vi "CurrentShiftCalc.vi"(8 "Date/Time":string, 9 "3rdShiftConfig":T1={"StartHour"=[{"Hour"=5, "Minute"=0}, {"Hour"=6, "Minute"=0}, {"Hour"=7, "Minute"=0}, {"Hour"=7, "Minute"=30}, {"Hour"=0, "Minute"=0}, {"Hour"=0, "Minute"=0}, {"Hour"=0, "Minute"=0}, {"Hour"=0, "Minute"=0}, {"Hour"=0, "Minute"=0}], "Goal"=[], "EndHour"=[{"Hour"=5, "Minute"=59}, {"Hour"=6, "Minute"=59}, {"Hour"=7, "Minute"=10}, {"Hour"=7, "Minute"=59}, {"Hour"=0, "Minute"=0}, {"Hour"=0, "Minute"=0}, {"Hour"=0, "Minute"=0}, {"Hour"=0, "Minute"=0}, {"Hour"=0, "Minute"=0}], "AM/PM"=[]} caption="3rdShift" {"AM/PM"."AM/PM" items=["AM", "PM"]; "EndHour"."Minute" items=["00", "1", "2", "3", "4", "5", "6", "7", "8", "9", "10", "11", "12", "13", "14", "15", "16", "17", "18", "19", "20", "21", "22", "23", "24", "25", "26", "27", "28", "29", "30", "31", "32", "33", "34", "35", "36", "37", "38", "39", "40", "41", "42", "43", "44", "45", "46", "47", "48", "49", "50", "51", "52", "53", "54", "55", "56", "57", "58", "59"]; "EndHour"."Hour" items=["0", "1", "2", "3", "4", "5", "6", "7", "8", "9", "10", "11", "12", "13", "14", "15", "16", "17", "18", "19", "20", "21", "22", "23"]; "StartHour"."Minute" items=["00", "1", "2", "3", "4", "5", "6", "7", "8", "9", "10", "11", "12", "13", "14", "15", "16", "17", "18", "19", "20", "21", "22", "23", "24", "25", "26", "27", "28", "29", "30", "31", "32", "33", "34", "35", "36", "37", "38", "39", "40", "41", "42", "43", "44", "45", "46", "47", "48", "49", "50", "51", "52", "53", "54", "55", "56", "57", "58", "59"]; "StartHour"."Hour" items=["0", "1", "2", "3", "4", "5", "6", "7", "8", "9", "10", "11", "12", "13", "14", "15", "16", "17", "18", "19", "20", "21", "22", "23"]}, 10 "2ndShiftConfig":T1={"StartHour"=[{"Hour"=5, "Minute"=0}, {"Hour"=6, "Minute"=0}, {"Hour"=7, "Minute"=0}, {"Hour"=7, "Minute"=30}, {"Hour"=0, "Minute"=0}, {"Hour"=0, "Minute"=0}, {"Hour"=0, "Minute"=0}, {"Hour"=0, "Minute"=0}, {"Hour"=0, "Minute"=0}], "Goal"=[], "EndHour"=[{"Hour"=5, "Minute"=59}, {"Hour"=6, "Minute"=59}, {"Hour"=7, "Minute"=10}, {"Hour"=7, "Minute"=59}, {"Hour"=0, "Minute"=0}, {"Hour"=0, "Minute"=0}, {"Hour"=0, "Minute"=0}, {"Hour"=0, "Minute"=0}, {"Hour"=0, "Minute"=0}], "AM/PM"=[{"AM/PM"=1}, {"AM/PM"=1}, {"AM/PM"=1}, {"AM/PM"=1}, {"AM/PM"=1}, {"AM/PM"=1}, {"AM/PM"=1}, {"AM/PM"=1}, {"AM/PM"=1}]} caption="2ndShift" {"AM/PM"."AM/PM" items=["AM", "PM"]; "EndHour"."Minute" items=["00", "1", "2", "3", "4", "5", "6", "7", "8", "9", "10", "11", "12", "13", "14", "15", "16", "17", "18", "19", "20", "21", "22", "23", "24", "25", "26", "27", "28", "29", "30", "31", "32", "33", "34", "35", "36", "37", "38", "39", "40", "41", "42", "43", "44", "45", "46", "47", "48", "49", "50", "51", "52", "53", "54", "55", "56", "57", "58", "59"]; "EndHour"."Hour" items=["00", "1", "2", "3", "4", "5", "6", "7", "8", "9", "10", "11", "12", "13", "14", "15", "16", "17", "18", "19", "20", "21", "22", "23"]; "StartHour"."Minute" items=["00", "1", "2", "3", "4", "5", "6", "7", "8", "9", "10", "11", "12", "13", "14", "15", "16", "17", "18", "19", "20", "21", "22", "23", "24", "25", "26", "27", "28", "29", "30", "31", "32", "33", "34", "35", "36", "37", "38", "39", "40", "41", "42", "43", "44", "45", "46", "47", "48", "49", "50", "51", "52", "53", "54", "55", "56", "57", "58", "59"]; "StartHour"."Hour" items=["0", "1", "2", "3", "4", "5", "6", "7", "8", "9", "10", "11", "12", "13", "14", "15", "16", "17", "18", "19", "20", "21", "22", "23"]}, 11 "1stShiftConfig":T1={"StartHour"=[{"Hour"=5, "Minute"=0}, {"Hour"=6, "Minute"=0}, {"Hour"=7, "Minute"=0}, {"Hour"=7, "Minute"=30}, {"Hour"=0, "Minute"=0}, {"Hour"=0, "Minute"=0}, {"Hour"=0, "Minute"=0}, {"Hour"=0, "Minute"=0}, {"Hour"=0, "Minute"=0}], "Goal"=[], "EndHour"=[{"Hour"=5, "Minute"=59}, {"Hour"=6, "Minute"=59}, {"Hour"=7, "Minute"=10}, {"Hour"=7, "Minute"=59}, {"Hour"=0, "Minute"=0}, {"Hour"=0, "Minute"=0}, {"Hour"=0, "Minute"=0}, {"Hour"=0, "Minute"=0}, {"Hour"=0, "Minute"=0}], "AM/PM"=[{"AM/PM"=0}, {"AM/PM"=0}, {"AM/PM"=0}, {"AM/PM"=0}, {"AM/PM"=0}, {"AM/PM"=0}, {"AM/PM"=0}, {"AM/PM"=0}, {"AM/PM"=0}]} caption="1stShift" {"AM/PM"."AM/PM" items=["AM", "PM"]; "EndHour"."Minute" items=["00", "1", "2", "3", "4", "5", "6", "7", "8", "9", "10", "11", "12", "13", "14", "15", "16", "17", "18", "19", "20", "21", "22", "23", "24", "25", "26", "27", "28", "29", "30", "31", "32", "33", "34", "35", "36", "37", "38", "39", "40", "41", "42", "43", "44", "45", "46", "47", "48", "49", "50", "51", "52", "53", "54", "55", "56", "57", "58", "59"]; "EndHour"."Hour" items=["0", "1", "2", "3", "4", "5", "6", "7", "8", "9", "10", "11", "12", "13", "14", "15", "16", "17", "18", "19", "20", "21", "22", "23"]; "StartHour"."Minute" items=["00", "1", "2", "3", "4", "5", "6", "7", "8", "9", "10", "11", "12", "13", "14", "15", "16", "17", "18", "19", "20", "21", "22", "23", "24", "25", "26", "27", "28", "29", "30", "31", "32", "33", "34", "35", "36", "37", "38", "39", "40", "41", "42", "43", "44", "45", "46", "47", "48", "49", "50", "51", "52", "53", "54", "55", "56", "57", "58", "59"]; "StartHour"."Hour" items=["0", "1", "2", "3", "4", "5", "6", "7", "8", "9", "10", "11", "12", "13", "14", "15", "16", "17", "18", "19", "20", "21", "22", "23"]}) -> (3 "Shift":string)   [LabVIEW 2017]
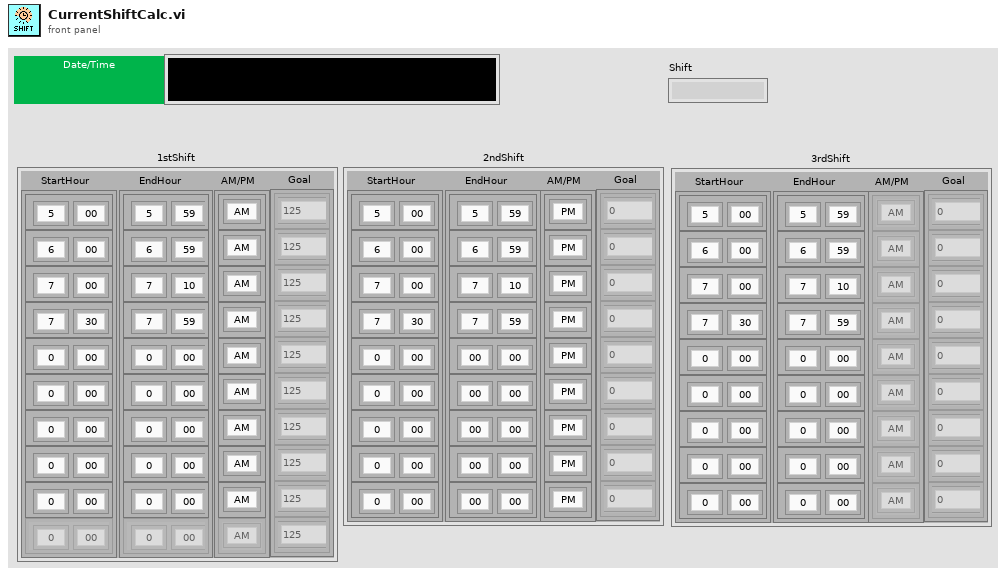
[diagram p1: front panel]
types:
  T1 = cluster{"StartHour":cluster{"Hour":u16, "Minute":u16}[], "Goal":cluster{"Goal":dbl}[], "EndHour":cluster{"Hour":u16, "Minute":u16}[], "AM/PM":cluster{"AM/PM":u16}[]}
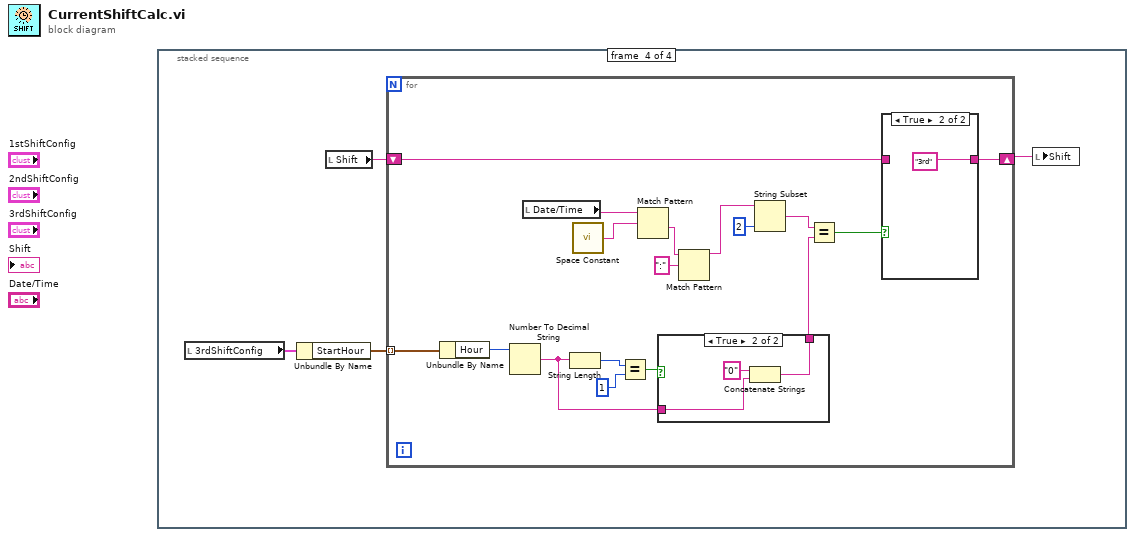
[diagram p0: block diagram]
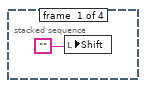
[diagram p2: hidden frame]
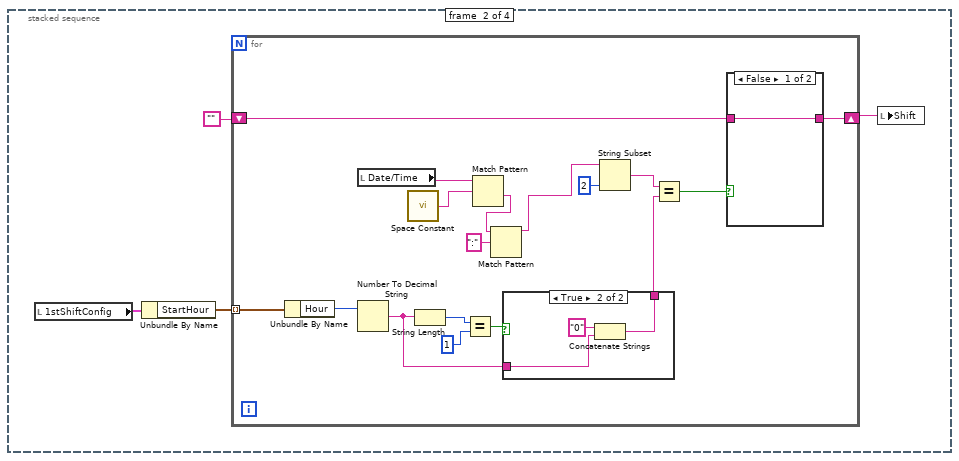
[diagram p3: hidden frame]
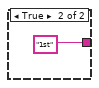
[diagram p5: hidden frame]
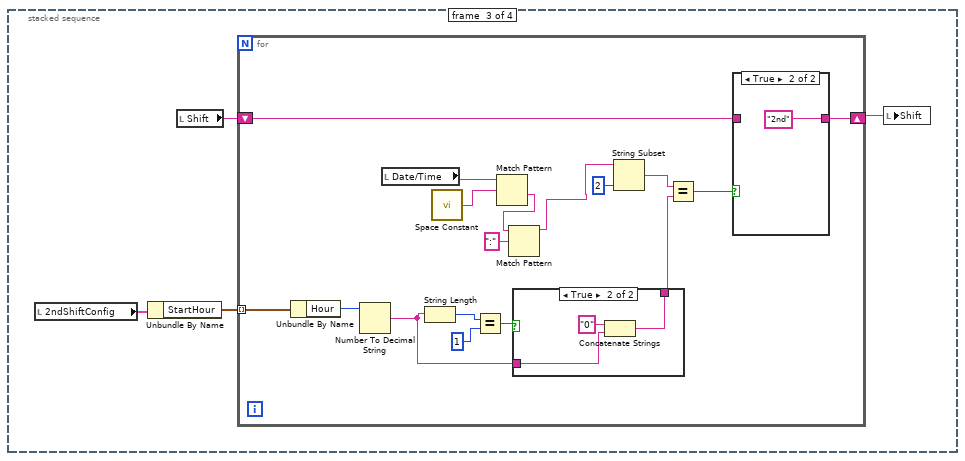
[diagram p6: hidden frame]
diagram:
  n1 = stacked-sequence {
    frame #0 {
      n2 = local write "Shift"("") -> ()
    }
    frame #1 {
      n3 = local read "1stShiftConfig"() -> (w5:T1)
      n4 = Unbundle By Name(w5) -> ("StartHour"=w4:cluster{"Hour":u16, "Minute":u16}[])
      n5 = for {
        tunnel: w4 -> [w19] mode=indexing
        shift-right: [w16] -> w3
        shift-left: "" -> [w17]
        n6 = Unbundle By Name(w19) -> ("Hour"=w12:u16)
        n7 = local read "Date/Time"() -> (w22:string)
        n8 = Number To Decimal String(number=w12) -> (decimal integer string=w7:string)  [unwired: 1 in]
        n9 = call <vilib>:"Space Constant.vi"() -> ("String"=w21:string)
        n10 = String Length(string=w7) -> (length=w10:i32)
        n11 = Equal?(x=w10, y=1) -> (x = y?=w8:bool)
        n12 = Match Pattern(string=w22, regular expression=w21) -> (after substring=w13:string)  [unwired: 1 in, 3 out]
        n13 = Match Pattern(string=w13, regular expression=":") -> (before substring=w14:string)  [unwired: 1 in, 3 out]
        n14 = case shown="True" w8 {
          tunnel: w7 -> [w23 w25]
          tunnel: [w23 w24] -> w6
          frame False {
          }
          frame True {
            n15 = Concatenate Strings("0" ("string"), w25) -> (w24:string)
          }
        }
        n16 = String Subset(string=w14, length (rest)=2 ("length (rest)")) -> (substring=w18:string)  [unwired: 1 in]
        n17 = Equal?(x=w18, y=w6) -> (x = y?=w11:bool)
        n18 = case shown="False" w11 {
          tunnel: w17 -> [w27 _]
          tunnel: [w27 "1st"] -> w16
          frame False {
          }
          frame True {
          }
        }
      }
      n19 = local write "Shift"(w3) -> ()
    }
    frame #2 {
      n20 = local read "2ndShiftConfig"() -> (w32:T1)
      n21 = Unbundle By Name(w32) -> ("StartHour"=w31:cluster{"Hour":u16, "Minute":u16}[])
      n22 = local read "Shift"() -> (w29:string)
      n23 = for {
        tunnel: w31 -> [w46] mode=indexing
        shift-right: [w43] -> w30
        shift-left: w29 -> [w44]
        n24 = Unbundle By Name(w46) -> ("Hour"=w39:u16)
        n25 = Number To Decimal String(number=w39) -> (decimal integer string=w34:string)  [unwired: 1 in]
        n26 = local read "Date/Time"() -> (w49:string)
        n27 = String Length(string=w34) -> (length=w37:i32)
        n28 = call <vilib>:"Space Constant.vi"() -> ("String"=w48:string)
        n29 = Equal?(x=w37, y=1) -> (x = y?=w35:bool)
        n30 = Match Pattern(string=w49, regular expression=w48) -> (after substring=w40:string)  [unwired: 1 in, 3 out]
        n31 = Match Pattern(string=w40, regular expression=":") -> (before substring=w41:string)  [unwired: 1 in, 3 out]
        n32 = case shown="True" w35 {
          tunnel: w34 -> [w50 w52]
          tunnel: [w50 w51] -> w33
          frame False {
          }
          frame True {
            n33 = Concatenate Strings("0" ("string"), w52) -> (w51:string)
          }
        }
        n34 = String Subset(string=w41, length (rest)=2 ("length (rest)")) -> (substring=w45:string)  [unwired: 1 in]
        n35 = Equal?(x=w45, y=w33) -> (x = y?=w38:bool)
        n36 = case shown="True" w38 {
          tunnel: w44 -> [w54 _]
          tunnel: [w54 "2nd"] -> w43
          frame False {
          }
          frame True {
          }
        }
      }
      n37 = local write "Shift"(w30) -> ()
    }
    frame #3 {
      n38 = local read "3rdShiftConfig"() -> (w59:T1)
      n39 = Unbundle By Name(w59) -> ("StartHour"=w58:cluster{"Hour":u16, "Minute":u16}[])
      n40 = local read "Shift"() -> (w56:string)
      n41 = for {
        tunnel: w58 -> [w73] mode=indexing
        shift-right: [w70] -> w57
        shift-left: w56 -> [w71]
        n42 = Unbundle By Name(w73) -> ("Hour"=w69:u16)
        n43 = Number To Decimal String(number=w69) -> (decimal integer string=w61:string)  [unwired: 1 in]
        n44 = local read "Date/Time"() -> (w76:string)
        n45 = String Length(string=w61) -> (length=w64:i32)
        n46 = call <vilib>:"Space Constant.vi"() -> ("String"=w75:string)
        n47 = Equal?(x=w64, y=1) -> (x = y?=w63:bool)
        n48 = Match Pattern(string=w76, regular expression=w75) -> (after substring=w66:string)  [unwired: 1 in, 3 out]
        n49 = case shown="True" w63 {
          tunnel: w61 -> [w77 w79]
          tunnel: [w77 w78] -> w60
          frame False {
          }
          frame True {
            n50 = Concatenate Strings("0" ("string"), w79) -> (w78:string)
          }
        }
        n51 = Match Pattern(string=w66, regular expression=":") -> (before substring=w67:string)  [unwired: 1 in, 3 out]
        n52 = String Subset(string=w67, length (rest)=2 ("length (rest)")) -> (substring=w72:string)  [unwired: 1 in]
        n53 = Equal?(x=w72, y=w60) -> (x = y?=w65:bool)
        n54 = case shown="True" w65 {
          tunnel: w71 -> [w81 _]
          tunnel: [w81 "3rd"] -> w70
          frame False {
          }
          frame True {
          }
        }
      }
      n55 = local write "Shift"(w57) -> ()
    }
  }
